vi "Read.vi"(8 "error in (no error)":errorcluster, 11 "String Array in":refnum<class "String Array.lvclass">) -> (0 "error out":errorcluster, 2 "String Array":string[](array[string]), 3 "String Array out":refnum<class "String Array.lvclass">)   [LabVIEW 2020, in "Data.lvlib" / "String Array.lvclass"]
doc: "Read String Array."
uses:
  String Array.lvclass
  String Array.lvclass/String Array.ctl
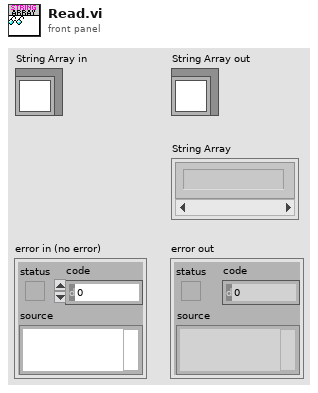
[diagram p1: front panel]
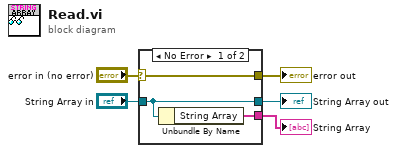
[diagram p0: block diagram]
diagram:
  n1 = case shown="No Error" "error in (no error)" {
    selector: "error in (no error)" -> [w8 w9]
    tunnel: [w8 w9] -> w4
    tunnel: [w7 w10] -> w2
    tunnel: "String Array in" -> [w7 w10]
    tunnel: [w6 _] -> w1
    frame No Error {
      n2 = Unbundle By Name(w7) -> ("String Array"=w6:string[])
    }
    frame Error {
    }
  }
  "error out" <- w4
  "String Array out" <- w2
  "String Array" <- w1
